vi "sub_strainx4_buf.vi"(7 "cmd":T1, 8 "error in":errorcluster, 11 "strain filter_n_nulling wf":waveform(dbl)[](array[waveform])) -> (0 "error out":errorcluster, 3 "queue out":refnum<queue>)   [LabVIEW 2016]
uses:
  ctl/Data_buf_cmd.ctl
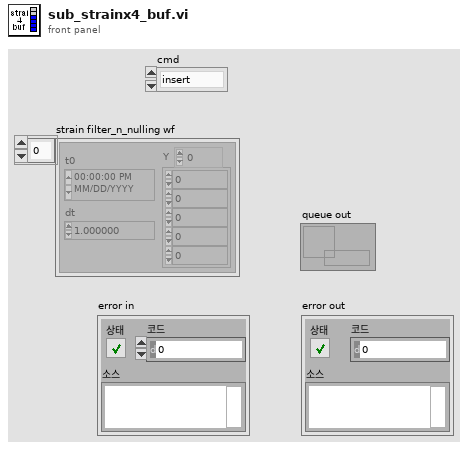
[diagram p1: front panel]
types:
  T1 = typedef "Data_buf_cmd.ctl" = enum16{"insert", "default", "create", "clear"}
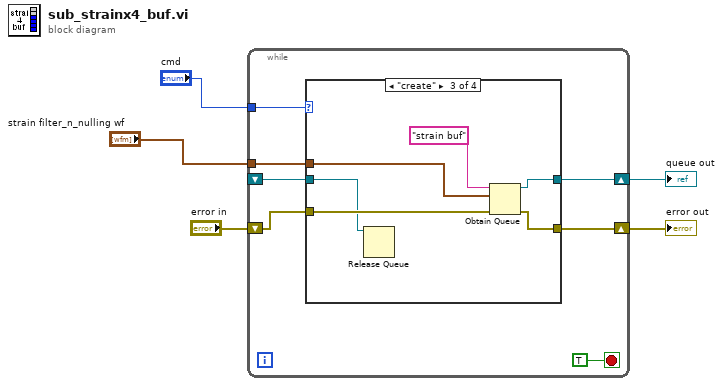
[diagram p0: block diagram]
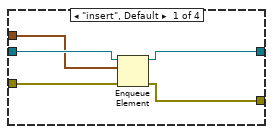
[diagram p2: hidden frame]
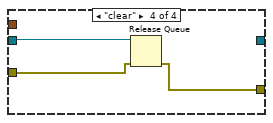
[diagram p4: hidden frame]
diagram:
  n1 = while {
    shift-right: [w9] -> w1
    shift-left: _ -> [w10]
    tunnel: "cmd" -> [w11]
    shift-right: [w7] -> w4
    shift-left: "error in" -> [w8]
    tunnel: "strain filter_n_nulling wf" -> [w6]
    stop <- TRUE stop-if-true
    n2 = case shown="\"create\"" w11 {
      tunnel: w10 -> [w17 w19 w20 w28]
      tunnel: [w16 w19 w25 _] -> w9
      tunnel: w8 -> [w15 w18 w24 w27]
      tunnel: [w14 w18 w23 w26] -> w7
      tunnel: w6 -> [w13 _ w22 _]
      frame "insert", Default {
        n3 = Enqueue Element(queue=w17, element=w13, error in (no error)=w15) -> (queue out=w16:refnum<queue>, error out=w14:errorcluster)  [unwired: 1 in, 1 out]
      }
      frame "default" {
      }
      frame "create" {
        n4 = Release Queue(queue=w20) -> ()  [unwired: 2 in, 3 out]
        n5 = Obtain Queue(name (unnamed)="strain buf" ("이름(이름없음)"), element data type=w22, error in (no error)=w24) -> (queue out=w25:refnum<queue>, error out=w23:errorcluster)  [unwired: 2 in, 1 out]
      }
      frame "clear" {
        n6 = Release Queue(queue=w28, error in (no error)=w27) -> (error out=w26:errorcluster)  [unwired: 1 in, 2 out]
      }
    }
  }
  "error out" <- w4
  "queue out" <- w1
